vi "DCC_Close.vi"(8 "Error In":errorcluster, 11 "DLL Path":path) -> (0 "Error Out":errorcluster)   [LabVIEW 2019]
doc: "This closing function closes all open references and closes the DLL reference in a proer way.\n\nAugust 2018\nFrank Quadt & Stefan Smietana\ninfo@becker-hickl.com"
panel:
  # "(c) 2021 Becker & Hickl GmbH\n     All Rights Reserved."
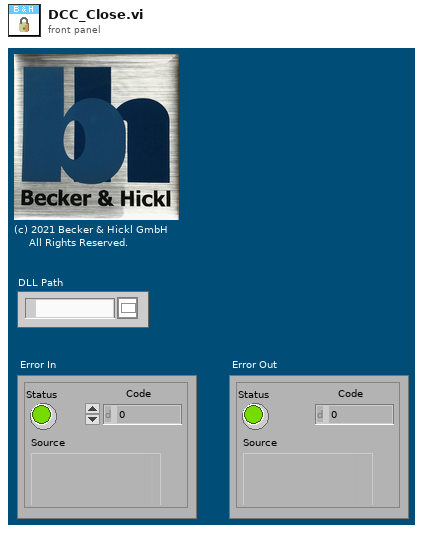
[diagram p1: front panel]
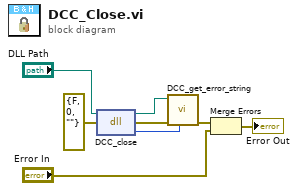
[diagram p0: block diagram]
diagram:
  n1 = dll-call lib="X:/FQ/DCC v.2.3/dll/dcc64.dll" fn="DCC_close"(path in="DLL Path", error in=errorcluster {"status"=FALSE, "code"=0, "source"=""} ("error constant")) -> (path out=w6:path, error out=w7:errorcluster, "return type"=w8:i16)  [unwired: 1 in]
  n2 = call "DCC_get_error_string.vi"("Error ID"=w8, "Error In"=w7, "DLL Path"=w6) -> ("Error Out"=w5:errorcluster)  [unwired: 6 in, 2 out]
  n3 = Merge Errors(w5, "Error In") -> (→"Error Out":errorcluster)
